vi "BeverageFlyweightFactory_Create.vi"(8 "Error In":errorcluster, 11 "reference in":refnum<class "BeverageFlyweightFactory.lvclass">) -> (0 "Error Out":errorcluster, 3 "reference out":refnum<class "BeverageFlyweightFactory.lvclass">)   [LabVIEW 2020, in "BeverageFlyweightFactory.lvclass"]
uses:
  BeverageFlyweightFactory.lvclass
  BeverageType.ctl
  IBeverage_interface/IBeverage.lvclass
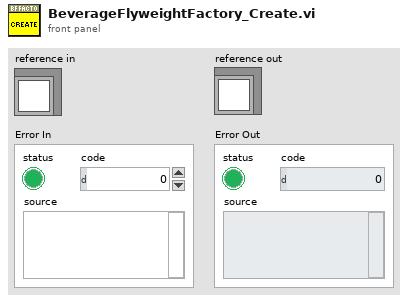
[diagram p1: front panel]
types:
  T1 = typedef "BeverageType.ctl" = enum16{"BubbleMilk", "FoamMilk", "OolongMilk", "CoconutMilk"}
  T2 = typedef "BeverageFlyweightFactory.lvclass/ObjectAttributes.ctl" = cluster{"_beverages":map{T1, refnum<class "IBeverage.lvclass">}}
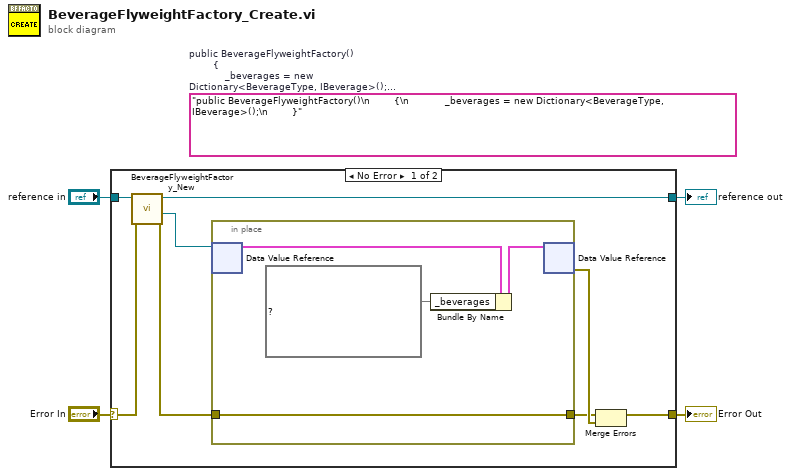
[diagram p0: block diagram]
diagram:
  (unwired) "public BeverageFlyweightFactory()\n        {\n            _beverages = new Dictionary<BeverageType, IBeverage>();\n        }"  # public BeverageFlyweightFactory()         {             _beverages = new Dictionary<BeverageType, IBeverage>();         }
  n1 = case shown="No Error" "Error In" {
    selector: "Error In" -> [w11 w18]
    tunnel: [w5 w18] -> w3
    tunnel: "reference in" -> [w12 w17]
    tunnel: [w10 w17] -> w1
    frame No Error {
      n2 = call "BeverageFlyweightFactory_New.vi"("error in (no error)"=w11, "reference in"=w12) -> ("error out"=w7:errorcluster, "DVRRefOut"=w8:refnum<data-value>, "reference out"=w10:refnum<class "BeverageFlyweightFactory.lvclass">)  [unwired: 6 in, 1 out]
      n3 = in-place {
        in-place-border: w7 -> [w14]
        in-place-border: [w14] -> w6
        n4 = in-place-dvr #1(w8) -> (w15:T2)  [unwired: 1 out]
        n5 = Bundle By Name(cluster=w15, "_beverages"=map{T1, refnum<class "IBeverage.lvclass">} {}) -> (w16:T2)
        n6 = in-place-dvr #1(w16) -> (w9:errorcluster)  [unwired: 1 out]
      }
      n7 = Merge Errors(w6, w9) -> (w5:errorcluster)
    }
    frame Error {
      # "VI-TechBaseTemplate_Simple_4x4x4"
    }
  }
  "Error Out" <- w3
  "reference out" <- w1
